vi "CAN_MotorControlandBMS.vi"(8 "error in (no error)":errorcluster) -> (0 "error out":errorcluster)   [LabVIEW 2018]
uses:
  BMS/OrionBMSClass.lvclass
  BMS/MotorControllerClass.lvclass
  <vilib>/Platform/TimedLoop/XDataNode/timing_clust.ctl
  <vilib>/Platform/TimedLoop/XDataNode/nitl_modes.ctl
  <vilib>/Platform/TimedLoop/XDataNode/wakeup.ctl
  Type_Def/TypeDef_BMSData.ctl
  Type_Def/TypeDef_BmsStatus.ctl
  Type_Def/Type_Def MotorControlState.ctl
  Type_Def/TypeDef_MotorData.ctl
  <vilib>/platform/TimedLoop/XDataNode/XDataNode.xnode
  <vilib>/Platform/TimedLoop/XDataNode/XDNodeRunTimeDep.lvlib
panel:
  out "stopDriveRes":u32
  out "changeTargetRes":u32
  out "startDriveRes":u32
  out "controlWord6Res":i16
  out "targetTorqueRes":u32
  out "BMS Freeze":bool
  out "Loop Counter":i32
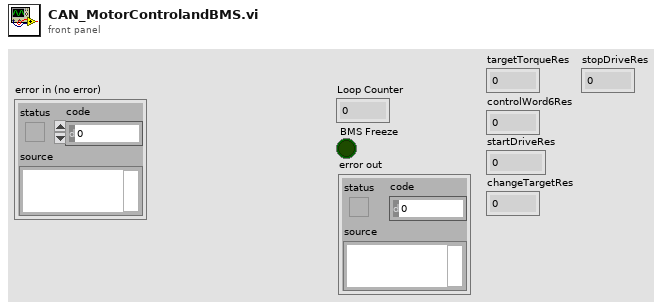
[diagram p1: front panel]
types:
  T1 = typedef "Type_Def MotorControlState.ctl" = enum16{"Idle", "Initialization", "Running", "Termination"}
  T2 = typedef "XDNodeRunTimeDep.lvlib/timing_clust.ctl" = cluster{"Expected End [f-1]":u64, "Actual End [f-1]":u64, "Finished Late? [f-1]":bool, "Expected End [i-1]":u64, "Actual End [i-1]":u64, "Finished Late? [i-1]":bool, "Expected Start [i]":u64, "Actual Start [i]":u64, "Expected Start [f]":u64, "Actual Start [f]":u64, "Source Name":string, "Structure Name":string, "Period":i64, "Deadline":i64, "Offset":i64, "Start":i64, "Priority":i32, "Timeout":i32, "Mode":T3, "Wakeup Reason":T4, "Error":errorcluster, "Source Type":string, "Secondary Source Type":string, "Global End Time":u64, "Global Start Time":u64, "Frame Duration":u64, "Iteration Duration":u64, "Assigned CPU":i32, "I/O Scan Engine Mode":u32}
  T3 = typedef "XDNodeRunTimeDep.lvlib/nitl_modes.ctl" = enum32{"No Change", "Process missed periods, maintain original phase", "Discard missed periods, maintain original phase", "Process missed periods, ignore original phase", "Discard missed periods, ignore original phase"}
  T4 = typedef "XDNodeRunTimeDep.lvlib/wakeup.ctl" = enum32{"Normal", "Aborted", "Asynchronous wakeup", "Timing source error", "Timed loop error", "Timeout"}
  T5 = typedef "TypeDef_BMSData.ctl" = cluster{"Max Cell Voltage (V)":dbl, "Max Cell ID":dbl, "Min Cell Voltage (V)":dbl, "Min Cell ID":dbl, "State of Charge (%)":dbl, "Average Voltage (V)":dbl, "Voltage Delta (V)":dbl, "Pack Current (A)":dbl, "Pack Voltage (V)":dbl, "Max Resistance (Ohm)":dbl, "Min Resistance (Ohm)":dbl, "Average Resistance (Ohm)":dbl, "Delta Resistance (Ohm)":dbl, "Highest Temperature(F)":dbl, "BmsStatus":T6}
  T6 = typedef "TypeDef_BmsStatus.ctl" = cluster{"isFault":bool, "isolationMonitoring":bool}
  T7 = typedef "TypeDef_MotorData.ctl" = cluster{" Velocity (RPM)":i32, " MotorTemp(C)":u8, " ControlTemp(C)":u8, " DcLinkVolt(V)":dbl, " ErrorCode":dbl, "IsAlive":bool, "motorStatus":cluster{"isReady":bool, "isOn":bool, "isOperEn":bool, "isFault":bool, "isVoltEn":bool, "targetReached":bool, "isWarning":bool}, "motorControllerState":u16}
  T8 = cluster{"error code":dbl, "error register":dbl, "manufacturer specific error field":dbl[]}
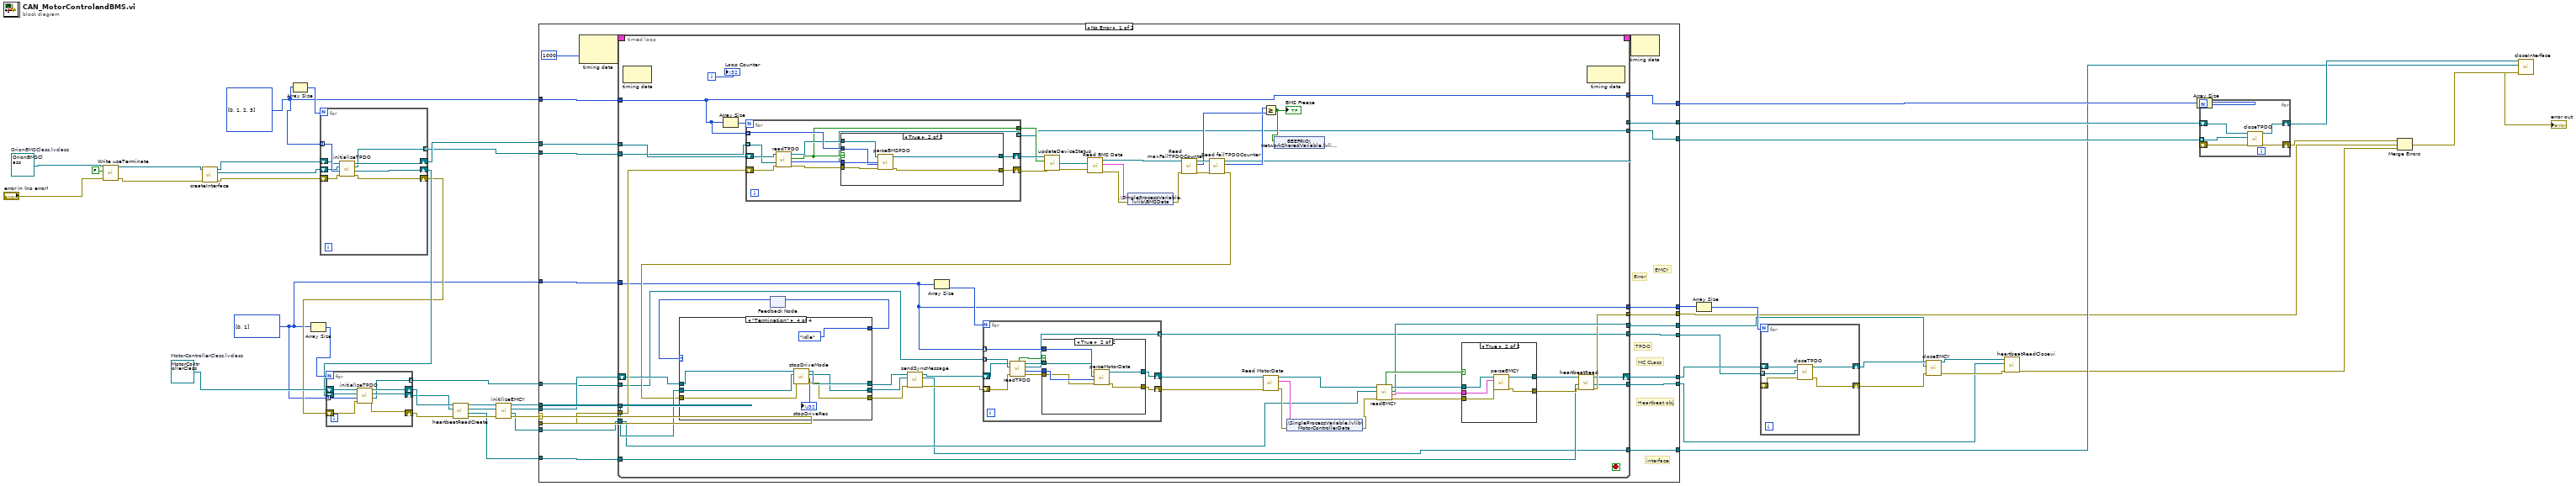
[diagram p0: block diagram]
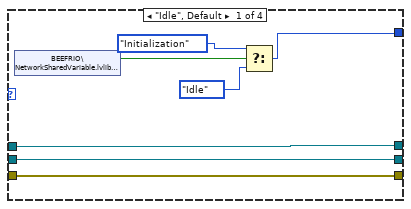
[diagram p4: hidden frame]
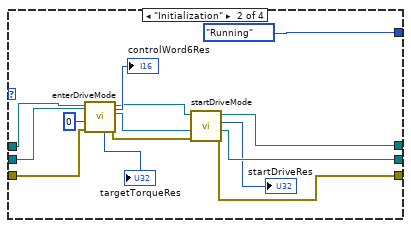
[diagram p5: hidden frame]
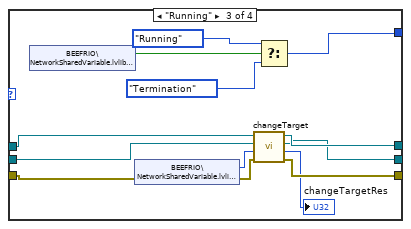
[diagram p6: hidden frame]
diagram:
  w20 = u8[] [0, 1] items=["PDO 1", "PDO 2", "PDO 3", "PDO 4"]
  w33 = refnum<class "MotorControllerClass.lvclass"> refnum  # MotorControllerClass.lvclass
  w41 = u8[] [0, 1, 2, 3] items=["PDO 1", "PDO 2", "PDO 3", "PDO 4"]
  w49 = refnum<class "OrionBMSClass.lvclass"> refnum  # OrionBMSClass.lvclass
  n1 = call-dynamic "Write useTerminate .vi"("error in (no error)"="error in (no error)", "useTerminate"=FALSE, "OrionBMS in"=w49) -> ("error out"=w46:errorcluster, "OrionBMS out"=w47:refnum<class "OrionBMSClass.lvclass">)  [unwired: 7 in]
  n2 = call "createInterface.vi"("error in (no error)"=w46, "OrionBMS in"=w47) -> ("error out"=w42:errorcluster, "interface object out"=w43:refnum<k20>, "OrionBMS out"=w44:refnum<class "OrionBMSClass.lvclass">)  [unwired: 7 in]
  n3 = Array Size(array=w41) -> (size(s)=w45:i32)
  n4 = Array Size(array=w20) -> (size(s)=w34:i32)
  n5 = for {
    N: w45 -> [_]
    tunnel: w41 -> [w58] mode=indexing
    shift-right: [w54] -> w40
    shift-left: w44 -> [w57]
    tunnel: [w51] -> w39 mode=indexing
    shift-right: [w53] -> w32
    shift-left: w43 -> [w56]
    shift-right: [w52] -> w31
    shift-left: w42 -> [w55]
    n6 = call "initializeTPDO.vi"("error in (no error)"=w55, "PDO channel"=w58, "interface object in"=w56, "OrionBMS in"=w57) -> ("error out"=w52:errorcluster, "interface object out"=w53:refnum<k20>, "TPDO object out"=w51:refnum<k20>, "OrionBMS out"=w54:refnum<class "OrionBMSClass.lvclass">)  [unwired: 2 in]
  }
  n7 = for {
    N: w34 -> [_]
    tunnel: w20 -> [w64] mode=indexing
    tunnel: [w61] -> w19 mode=indexing
    shift-right: [w63] -> w30
    shift-left: w33 -> [w66]
    shift-right: [w62] -> w29
    shift-left: w32 -> [w65]
    shift-right: [w60] -> w28
    shift-left: w31 -> [w59]
    n8 = call "initializeTPDO.vi"("error in (no error)"=w59, "PDO channel"=w64, "interface object in"=w65, "MotorControllerClass in"=w66) -> ("error out"=w60:errorcluster, "TPDO object out"=w61:refnum<k20>, "interface object out"=w62:refnum<k20>, "MotorControllerClass out"=w63:refnum<class "MotorControllerClass.lvclass">)  [unwired: 4 in]
  }
  n9 = call "heartbeatReadCreate.vi"("error in (no error)"=w28, "interface object in"=w29, "MotorControllerClass in"=w30) -> ("error out"=w25:errorcluster, "heartbeat object out"=w24:refnum<k20>, "interface object out"=w26:refnum<k20>, "MotorControllerClass out"=w27:refnum<class "MotorControllerClass.lvclass">)  [unwired: 5 in]
  n10 = call "initilizeEMCY.vi"("error in (no error)"=w25, "interface object in"=w26, "MotorControllerClass in"=w27) -> ("error out"=w23:errorcluster, "emergency object out"=w15:refnum<k20>, "interface object out"=w21:refnum<k20>, "MotorControllerClass out"=w22:refnum<class "MotorControllerClass.lvclass">)  [unwired: 5 in]
  n11 = case shown="No Error" w23 {
    selector: w23 -> [_ w243]
    tunnel: w41 -> [w86 w247]
    tunnel: w40 -> [w85 w245]
    tunnel: w39 -> [w84 w246]
    tunnel: [w77 w247] -> w17
    tunnel: [w76 w246] -> w37
    tunnel: w24 -> [w83 w239]
    tunnel: w23 -> [w82 _]
    tunnel: w22 -> [w81 w240]
    tunnel: w21 -> [w80 w238]
    tunnel: w20 -> [w79 w244]
    tunnel: w19 -> [w78 w241]
    tunnel: [w75 w245] -> w16
    tunnel: [w74 w239] -> w5
    tunnel: [w68 w242] -> w8
    tunnel: [w73 w243] -> w1
    tunnel: [w72 w244] -> w14
    tunnel: [w71 w240] -> w12
    tunnel: [w69 w241] -> w11
    tunnel: [w70 w238] -> w4
    tunnel: w15 -> [w67 w242]
    frame No Error {
      # "EMCY"
      # "Error"
      # "TPDO"
      # "MC CLass"
      # "interface"
      # "Heartbeat obj"
      n12 = node-c288(i64 1000 ("Period")) -> (w89:T2)  [unwired: 1 in]
      n13 = timed-loop {
        timing: w89 -> [_]
        timing-out: [_] -> w88
        tunnel: w86 -> [w126]
        tunnel: w85 -> [w142]
        tunnel: w84 -> [w141]
        tunnel: [w126] -> w77
        tunnel: [w125] -> w76
        tunnel: w83 -> [w96]
        tunnel: w82 -> [w122]
        tunnel: w80 -> [w120]
        tunnel: w67 -> [w106]
        tunnel: w79 -> [w93]
        tunnel: w78 -> [w114]
        tunnel: [w104] -> w75
        tunnel: [w99] -> w68
        tunnel: [w95] -> w73
        tunnel: [w94] -> w74
        tunnel: [w93] -> w72
        shift-right: [w92] -> w71
        shift-left: w81 -> [w121]
        tunnel: [w91] -> w69
        tunnel: [w90] -> w70
        i -> [w144]
        stop <- _ stop-if-true
        n14 = node-c288() -> ()  [unwired: 1 in, 1 out]
        n15 = Array Size(array=w126) -> (size(s)=w143:i32)
        n16 = for {
          N: w143 -> [_]
          tunnel: w141 -> [w222] mode=indexing
          tunnel: w126 -> [w219] mode=indexing
          tunnel: [w217] -> w139
          shift-right: [w216] -> w140
          shift-left: w142 -> [w223]
          shift-right: [w214] -> w138
          shift-left: w122 -> [w215]
          tunnel: [w213] -> w125 mode=indexing
          n17 = call "readTPDO.vi"("OrionBMS.lvclass"=w223, "TPDO object in"=w222, "error in (no error)"=w215) -> ("new data?"=w217:bool, "OrionBMS.lvclass"=w218:refnum<class "OrionBMSClass.lvclass">, "TPDO data"=w221:u8[], "TPDO object out"=w213:refnum<k20>, "error out"=w220:errorcluster)  [unwired: 3 in]
          n18 = case shown="True" w217 {
            tunnel: w221 -> [_ w231]
            tunnel: w220 -> [w224 w230]
            tunnel: w219 -> [_ w229]
            tunnel: w218 -> [w225 w228]
            tunnel: [w225 w227] -> w216
            tunnel: [w224 w226] -> w214
            frame False {
            }
            frame True {
              n19 = call "parseBMSPDO.vi"("error in (no error)"=w230, "PDO channel"=w229, "TPDO data"=w231, "OrionBMS in"=w228) -> ("error out"=w226:errorcluster, "OrionBMS out"=w227:refnum<class "OrionBMSClass.lvclass">)  [unwired: 6 in]
            }
          }
        }
        n20 = feedback #1() -> (w123:T1)  [unwired: 1 in]
        n21 = Array Size(array=w93) -> (size(s)=w115:i32)
        n22 = call "updateDeviceStatus.vi"("OrionBMS in"=w140, "isNewData"=w139, "error in (no error)"=w138) -> ("OrionBMS out"=w137:refnum<class "OrionBMSClass.lvclass">, "error out"=w136:errorcluster)  [unwired: 6 in]
        n23 = call-dynamic "Read BMS Data.vi"("error in (no error)"=w136, "OrionBMS in"=w137) -> ("error out"=w134:errorcluster, "BMS Data"=w135:T5, "OrionBMS out"=w131:refnum<class "OrionBMSClass.lvclass">)  [unwired: 7 in]
        n24 = shared-variable ".\\SingleProcessVariable.lvlib\\BMSData"(w135, error in=w134) -> (error out=w133:errorcluster)
        n25 = call-dynamic "Read maxFailTPDOCounter.vi"("error in (no error)"=w133, "OrionBMS in"=w131) -> ("error out"=w132:errorcluster, "maxFailTPDOCounter"=w129:u8, "OrionBMS out"=w130:refnum<class "OrionBMSClass.lvclass">)  [unwired: 7 in]
        n26 = call-dynamic "Read failTPDOCounter.vi"("error in (no error)"=w132, "OrionBMS in"=w130) -> ("error out"=w119:errorcluster, "failTPDOCounter"=w128:u8, "OrionBMS out"=w104:refnum<class "OrionBMSClass.lvclass">)  [unwired: 7 in]
        n27 = case shown="\"Termination\"" w123 {
          tunnel: [w176 Type_Def_MotorControlState."Running" ("Enum") w200 Type_Def_MotorControlState."Idle" ("Enum")] -> w124
          tunnel: [w175 w180 w195 w208] -> w118
          tunnel: w121 -> [w175 w187 w198 w211]
          tunnel: [w174 w181 w194 w207] -> w117
          tunnel: w120 -> [w174 w188 w197 w210]
          tunnel: w119 -> [w173 w186 w204 w209]
          tunnel: [w173 w178 w193 w206] -> w116
          frame "Idle", Default {
            n28 = shared-variable "BEEFRIO\\NetworkSharedVariable.lvlib\\driveEnable"() -> (w177:bool)  [unwired: 1 in, 1 out]
            n29 = Select(t=Type_Def_MotorControlState."Initialization" ("Enum"), s=w177, f=Type_Def_MotorControlState."Idle" ("Enum")) -> (s? t:f=w176:T1)
          }
          frame "Initialization" {
            n30 = call "enterDriveMode.vi"("error in (no error)"=w186, "targetNumber"=i16 0, "interface object in"=w188, "MotorControllerClass in"=w187) -> ("error out"=w182:errorcluster, "interface object out"=w183:refnum<k20>, "MotorControllerClass out"=w184:refnum<class "MotorControllerClass.lvclass">, "targetTorqueRes"=→"targetTorqueRes":u32, "controlWord6Res"=→"controlWord6Res":i16)  [unwired: 3 in]
            n31 = call "startDriveMode.vi"("error in (no error)"=w182, "interface object in"=w183, "MotorControllerClass in"=w184) -> ("error out"=w178:errorcluster, "interface object out"=w181:refnum<k20>, "startDriveRes"=→"startDriveRes":u32, "MotorControllerClass out"=w180:refnum<class "MotorControllerClass.lvclass">)  [unwired: 5 in]
          }
          frame "Running" {
            n32 = shared-variable "BEEFRIO\\NetworkSharedVariable.lvlib\\driveEnable"() -> (w203:bool)  [unwired: 1 in, 1 out]
            n33 = shared-variable "BEEFRIO\\NetworkSharedVariable.lvlib\\driveTarget"(error in=w204) -> (w199:i16, error out=w196:errorcluster)
            n34 = call "changeTarget.vi"("error in (no error)"=w196, "targetNumber"=w199, "interface object in"=w197, "MotorControllerClass in"=w198) -> ("error out"=w193:errorcluster, "changeTargetRes"=→"changeTargetRes":u32, "interface object out"=w194:refnum<k20>, "MotorControllerClass out"=w195:refnum<class "MotorControllerClass.lvclass">)  [unwired: 4 in]
            n35 = Select(t=Type_Def_MotorControlState."Running" ("Enum"), s=w203, f=Type_Def_MotorControlState."Termination" ("Enum")) -> (s? t:f=w200:T1)
          }
          frame "Termination" {
            n36 = call "stopDriveMode.vi"("error in (no error)"=w209, "interface object in"=w210, "MotorControllerClass in"=w211) -> ("error out"=w206:errorcluster, "stopDriveRes"=→"stopDriveRes":u32, "interface object out"=w207:refnum<k20>, "MotorControllerClass out"=w208:refnum<class "MotorControllerClass.lvclass">)  [unwired: 5 in]
          }
        }
        n37 = feedback-in #1(w124) -> ()
        n38 = call "sendSyncMessage.vi"("error in (no error)"=w116, "interface object in"=w117, "MotorControllerClass in"=w118) -> ("error out"=w112:errorcluster, "interface object out"=w90:refnum<k20>, "MotorControllerClass out"=w113:refnum<class "MotorControllerClass.lvclass">)  [unwired: 6 in]
        n39 = for {
          N: w115 -> [_]
          tunnel: w93 -> [w155] mode=indexing
          tunnel: w114 -> [w162] mode=indexing
          shift-right: [w154] -> w111
          shift-left: w113 -> [w161]
          shift-right: [w153] -> w110
          shift-left: w112 -> [w160]
          tunnel: [w152] -> w91 mode=indexing
          n40 = call "readTPDO.vi"("error in (no error)"=w160, "TPDO object in"=w162, "MotorControllerClass in"=w161) -> ("error out"=w157:errorcluster, "TPDO data"=w158:u8[], "TPDO object out"=w152:refnum<k20>, "MotorControllerClass out"=w156:refnum<class "MotorControllerClass.lvclass">, "new data?"=w159:bool)  [unwired: 4 in]
          n41 = case shown="True" w159 {
            tunnel: w158 -> [_ w168]
            tunnel: w157 -> [w163 w167]
            tunnel: w156 -> [w164 w169]
            tunnel: w155 -> [_ w170]
            tunnel: [w164 w166] -> w154
            tunnel: [w163 w165] -> w153
            frame False {
            }
            frame True {
              n42 = call "parseMotorData.vi"("error in (no error)"=w167, "TPDO data"=w168, "PDO channel"=w170, "MotorControllerClass in"=w169) -> ("error out"=w165:errorcluster, "MotorControllerClass out"=w166:refnum<class "MotorControllerClass.lvclass">)  [unwired: 6 in]
            }
          }
        }
        n43 = call-dynamic "Read MotorData.vi"("error in (no error)"=w110, "MotorControllerClass in"=w111) -> ("error out"=w108:errorcluster, "MotorData"=w109:T7, "MotorControllerClass out"=w107:refnum<class "MotorControllerClass.lvclass">)  [unwired: 7 in]
        n44 = Greater Or Equal?(x=w128, y=w129) -> (x >= y?=w127:bool)
        "BMS Freeze" <- w127
        n45 = shared-variable "BEEFRIO\\NetworkSharedVariable.lvlib\\BMSFreeze"(w127) -> ()  [unwired: 1 in, 1 out]
        n46 = shared-variable ".\\SingleProcessVariable.lvlib\\MotorControllerData"(w109, error in=w108) -> (error out=w105:errorcluster)
        n47 = call "readEMCY.vi"("error in (no error)"=w105, "emergency object in"=w106, "MotorControllerClass in"=w107) -> ("error out"=w100:errorcluster, "emergency message"=w101:T8, "emergency object out"=w99:refnum<k20>, "MotorControllerClass out"=w102:refnum<class "MotorControllerClass.lvclass">, "isNewMessage"=w103:bool)  [unwired: 4 in]
        n48 = case shown="True" w103 {
          tunnel: w102 -> [w146 w151]
          tunnel: w101 -> [_ w150]
          tunnel: w100 -> [w145 w149]
          tunnel: [w146 w148] -> w98
          tunnel: [w145 w147] -> w97
          frame False {
          }
          frame True {
            n49 = call "parseEMCY.vi"("error in (no error)"=w149, "emergency message"=w150, "MotorControllerClass in"=w151) -> ("error out"=w147:errorcluster, "MotorControllerClass out"=w148:refnum<class "MotorControllerClass.lvclass">)  [unwired: 7 in]
          }
        }
        n50 = call "heartbeatRead.vi"("error in (no error)"=w97, "heartbeat object in"=w96, "MotorControllerClass in"=w98) -> ("error out"=w95:errorcluster, "heartbeat object out"=w94:refnum<k20>, "MotorControllerClass out"=w92:refnum<class "MotorControllerClass.lvclass">)  [unwired: 6 in]
        n51 = node-c288() -> ()  [unwired: 1 in, 1 out]
        "Loop Counter" <- w144
      }
      n52 = node-c288(w88) -> ()  [unwired: 1 out]
    }
    frame Error {
    }
  }
  n53 = Array Size(array=w14) -> (size(s)=w13:i32)
  n54 = for {
    N: w13 -> [_]
    tunnel: w11 -> [w251] mode=indexing
    shift-right: [w249] -> w9
    shift-left: _ -> [w250]
    shift-right: [w248] -> w10
    shift-left: w12 -> [w252]
    n55 = call "closeTPDO.vi"("error in (no error)"=w250, "TPDO object in"=w251, "MotorControllerClass in"=w252) -> ("error out"=w249:errorcluster, "MotorControllerClass out"=w248:refnum<class "MotorControllerClass.lvclass">)  [unwired: 7 in]
  }
  n56 = call "closeEMCY.vi"("error in (no error)"=w9, "emergency object in"=w8, "MotorControllerClass in"=w10) -> ("error out"=w6:errorcluster, "MotorControllerClass out"=w7:refnum<class "MotorControllerClass.lvclass">)  [unwired: 7 in]
  n57 = call "heartbeatReadClosevi.vi"("error in (no error)"=w6, "heartbeat object in"=w5, "MotorControllerClass in"=w7) -> ("error out"=w3:errorcluster)  [unwired: 7 in, 1 out]
  n58 = Array Size(array=w17) -> (size(s)=w38:i32)
  n59 = for {
    N: w38 -> [_]
    tunnel: w37 -> [w255] mode=indexing
    shift-right: [w254] -> w36
    shift-left: w16 -> [w257]
    shift-right: [w253] -> w2
    shift-left: _ -> [w256]
    n60 = call "closeTPDO.vi"("error in (no error)"=w256, "TPDO object in"=w255, "OrionBMSClass in"=w257) -> ("error in (no error) 2"=w253:errorcluster, "OrionBMSClass out"=w254:refnum<class "OrionBMSClass.lvclass">)  [unwired: 7 in]
  }
  n61 = Merge Errors(w2, w1, w3) -> (w18:errorcluster)
  n62 = call "closeInterface.vi"("error in (no error)"=w18, "interface object in"=w4, "OrionBMS.lvclass"=w36) -> ("error out"=→"error out":errorcluster)  [unwired: 5 in, 1 out]
